vi "Bo Peep Auton.vi"() -> ()   [LabVIEW 2014]
uses:
  <vilib>/Rock Robotics/WPI/Solenoid/WPI_SolenoidValue.ctl
  <vilib>/Rock Robotics/WPI/Ultrasonic/WPI_SonarMB1010AnalogRefNum Registry Get.vi
  <vilib>/Rock Robotics/WPI/Ultrasonic/WPI_SonarMB1010AnalogGetRange.vi
  Robot Global Data.vi
  <vilib>/Rock Robotics/WPI/Solenoid/WPI_SolenoidSetEnum.vi
  <vilib>/Rock Robotics/WPI/RobotDrive/WPI_RobotDriveGetSetRefNum.vi
  <vilib>/Rock Robotics/WPI/RobotDrive/WPI_RobotDriveMecanumDrive_Cartesian.vi
panel:
  in  "Test":bool
  in  "Force state bo peep":i8
  out "Result":dbl(graph)
  out "result":dbl
  out "Destination":dbl
  out "Side Distance":dbl(graph)
  out "Front Distance":dbl(graph)
  out "Back Distance":dbl(graph)
  out "Bin Counter":i8
  out "Move?":bool
  out "Last State":i8
  out "State":i8
  out "Back Distance":dbl
  out "Front Distance":dbl
  out "Side Distance":dbl
  out "Bin found?":bool
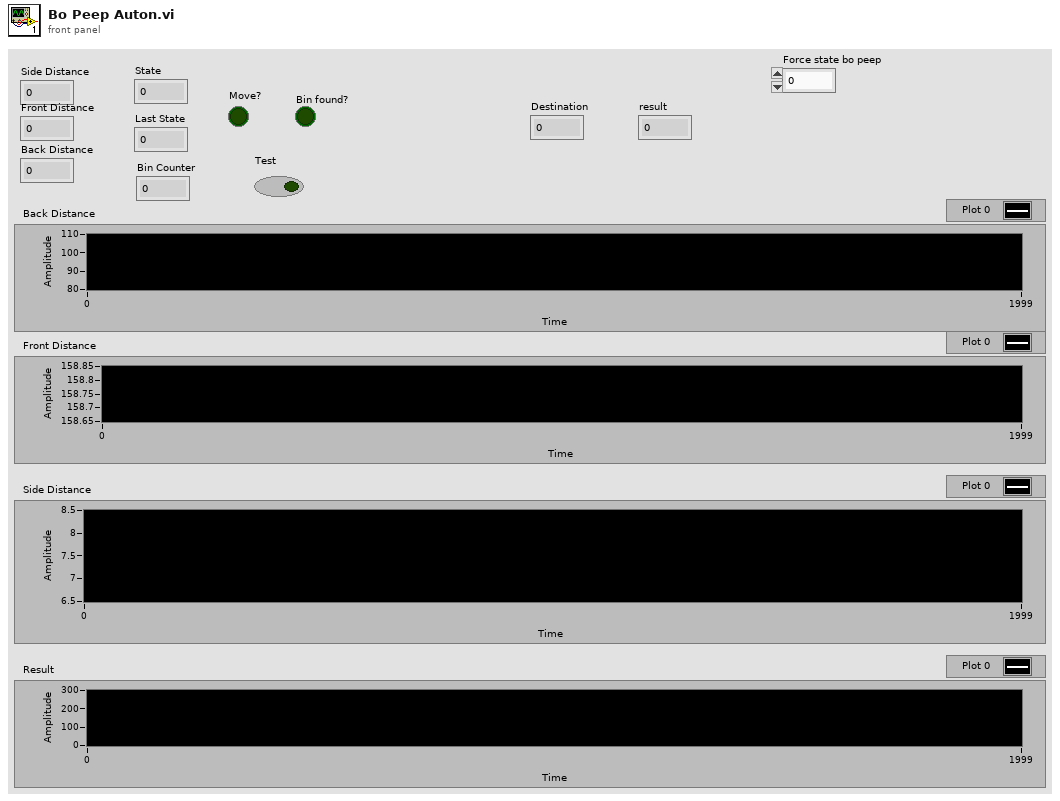
[diagram p1: front panel]
types:
  T1 = typedef "WPI_SonarMB1010AnalogDeviceRef.ctl" = cluster{"AIDeviceRef":T2, "Scaling factor (V/in)":dbl, "Average Bits":u8}
  T2 = typedef "WPI_AnalogChannelDevRef.ctl" = cluster{"DevStatus":errorcluster, "Controller":T3, "Analog Channel":T4}
  T3 = typedef "FPGA_TypedefAnalogModule.ctl" = enum16{"Controller 1"}
  T4 = typedef "FPGA_AIChannel.ctl" = enum8{"AI 0", "AI 1", "AI 2", "AI 3", "AI MXP 0", "AI MXP 1", "AI MXP 2", "AI MXP 3", "Invalid"}
  T5 = typedef "WPI_SolenoidValue.ctl" = enum16{"Off", "On", "Forward", "Reverse"}
  T6 = typedef "WPI_ServoDeviceRef.ctl" = cluster{"DeviceStatus":errorcluster, "Controller":T7, "PWM Channel":T8, "DeadBand":T9}
  T7 = typedef "FPGA_TypedefDigitalModule.ctl" = enum16{"Controller 1"}
  T8 = typedef "FPGA_DIOPWMChannel.ctl" = enum8{"PWM 0", "PWM 1", "PWM 2", "PWM 3", "PWM 4", "PWM 5", "PWM 6", "PWM 7", "PWM 8", "PWM 9", "PWM MXP 0", "PWM MXP 1", "PWM MXP 2", "PWM MXP 3", "PWM MXP 4", "PWM MXP 5", "PWM MXP 6", "PWM MXP 7", "PWM MXP 8", "PWM MXP 9", "Invalid"}
  T9 = typedef "WPI_PWMDeadband.ctl" = cluster{"Name":string, "maxPositivePwm":i32, "minPositivePwm":i32, "centerPwm":i32, "maxNegativePwm":i32, "minNegativePwm":i32, "angularRange":u16}
  T10 = typedef "WPI_MotorControlDeviceRef.ctl" = cluster{"DeviceStatus":errorcluster, "Type":T11, "PWM":cluster{"Controller":T7, "PWM Channel":T8, "DeadBand":T9}, "CAN":cluster{"Device Number":u8, "Control Mode":T12, "Semaphore":T13, "Max Vout":dbl, "TalonSRX Control Mode":T14}, "Invert":bool, "TransformRef":T15, "InvTransformRef":T15}
  T11 = typedef "WPI_MotorControlType.ctl" = enum16{"PWM", "CAN", "CANTalonSRX"}
  T12 = typedef "WPI_CANJaguar_ControlMode.ctl" = enum8{"Percent VBus", "Current", "Speed", "Position", "Voltage"}
  T13 = typedef "Semaphore RefNum" = refnum<k1>
  T14 = typedef "WPI_CANTalonSRX_APIControlMode.ctl" = enum8{"Percent VBus", "Speed", "Position", "Slave", "Unchanged / Invalid"}
  T15 = typedef "WPI_PWMTransform_ConPane.ctl" = refnum<vi>
  T16 = typedef "WPI_SolenoidDevRef.ctl" = cluster{"DevStatus":errorcluster, "Pneumatics Control Module":u8, "Forward Solenoid Channel":T17, "Reverse Solenoid Channel":T17}
  T17 = typedef "WPI_SolenoidChannel.ctl" = enum8{"Solenoid 0", "Solenoid 1", "Solenoid 2", "Solenoid 3", "Solenoid 4", "Solenoid 5", "Solenoid 6", "Solenoid 7", "Invalid"}
  T18 = typedef "WPI_CANTalonSRX_GlobalStatus.ctl" = cluster{"Applied Throttle":dbl, "Module Enabled":bool, "CAN Error":errorcluster, "Closed Loop Error":dbl, "Forward Limit Switch Closed":bool, "Reverse Limit Switch Closed":bool, "Sensor Position":dbl, "Sensor Velocity":dbl, "Current":dbl, "Sticky Fault - Over Temp":bool, "Sticky Fault - Under Voltage":bool, "Sticky Fault - Forward Limit":bool, "Sticky Fault - Reverse Limit":bool, "Sticky Fault - Forward Soft Limit":bool, "Sticky Fault - Reverse Soft Limit":bool, "Brake is Enabled":bool, "Encoder Position":dbl, "Encoder Velocity":dbl, "Encoder Index Count":dbl, "Encoder A Pin State":bool, "Encoder B Pin State":bool, "Encoder Index Pin State":bool, "Analog In":dbl, "Analog In Velocity":dbl, "Temperature (C)":dbl, "Battery Voltage":dbl}
  T19 = typedef "WPI_DigitalInputDevRef.ctl" = cluster{"DevStatus":errorcluster, "DIO Channel":T20, "Controller":T7}
  T20 = typedef "FPGA_DIOChannel.ctl" = enum8{"DIO 0", "DIO 1", "DIO 2", "DIO 3", "DIO 4", "DIO 5", "DIO 6", "DIO 7", "DIO 8", "DIO 9", "DIO MXP 0", "DIO MXP 1", "DIO MXP 2", "DIO MXP 3", "DIO MXP 4", "DIO MXP 5", "DIO MXP 6", "DIO MXP 7", "DIO MXP 8", "DIO MXP 9", "DIO MXP 10", "DIO MXP 11", "DIO MXP 12", "DIO MXP 13", "DIO MXP 14", "DIO MXP 15", "Invalid"}
  T21 = typedef "WPI_DigitalOutputDevRef.ctl" = cluster{"Controller":T7, "DIO Channel":T20, "DevStatus":errorcluster}
  T22 = typedef "WPI_RobotDriveDevRef.ctl" = cluster{"DevStatus":errorcluster, "Motors[]":T10[], "Square Inputs":bool, "Max Output":dbl}
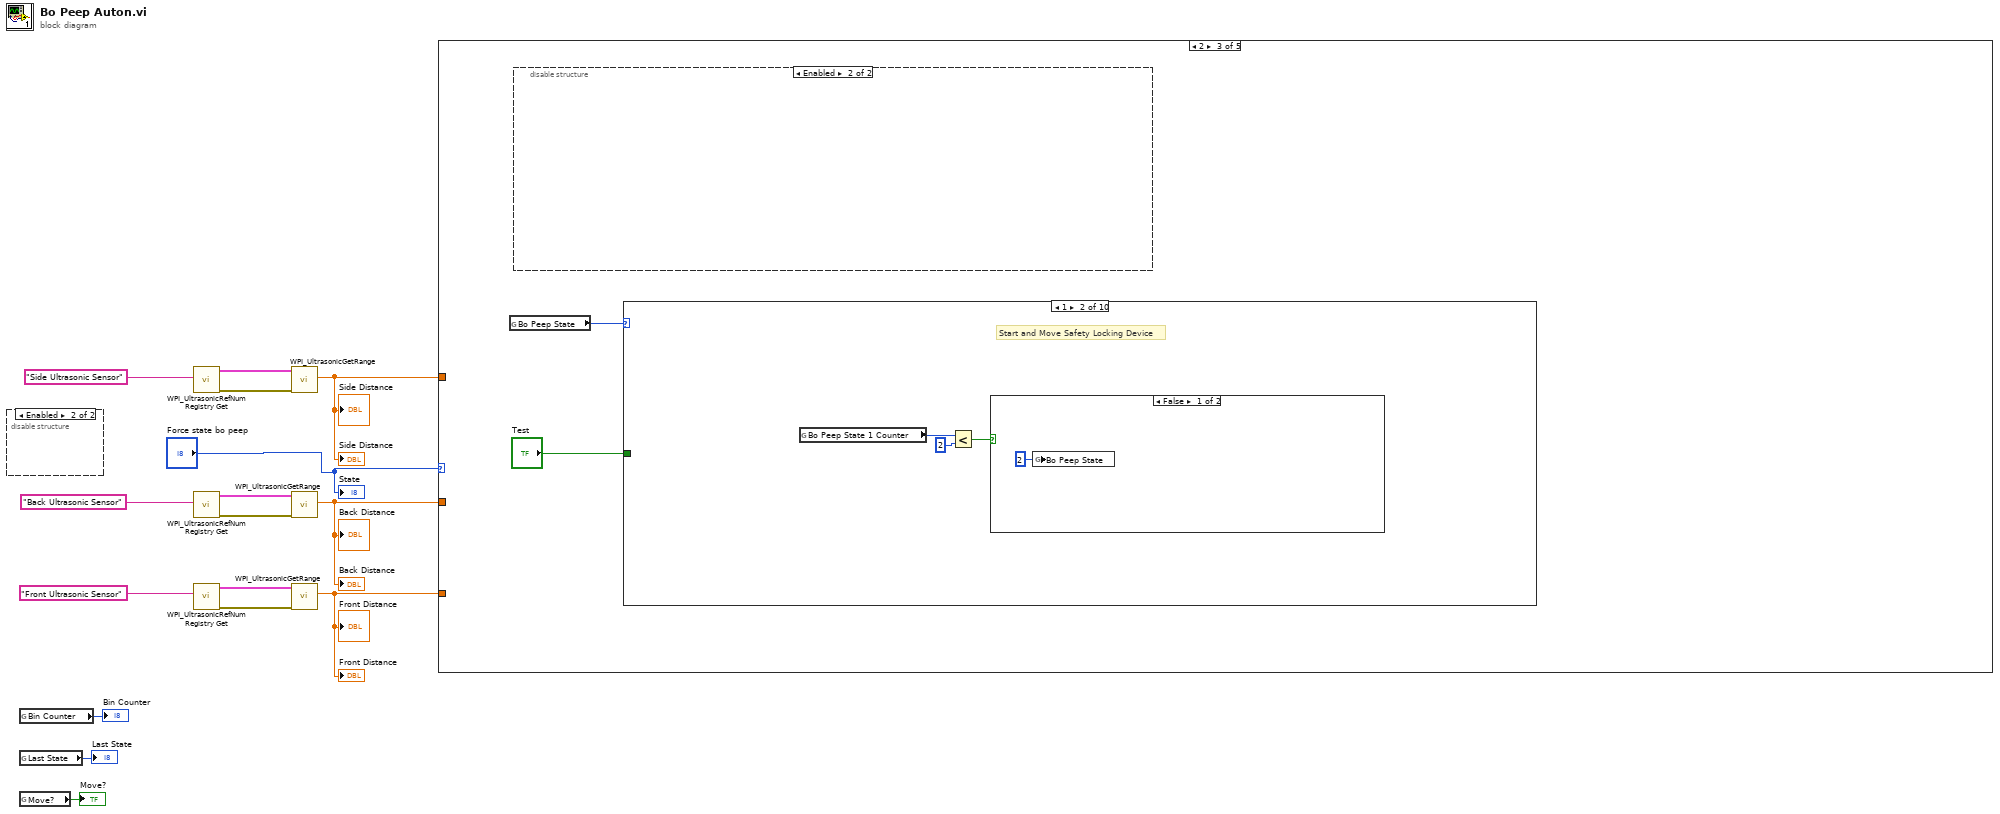
[diagram p0: block diagram]
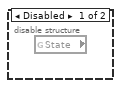
[diagram p2: hidden frame]
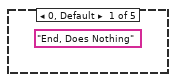
[diagram p3: hidden frame]
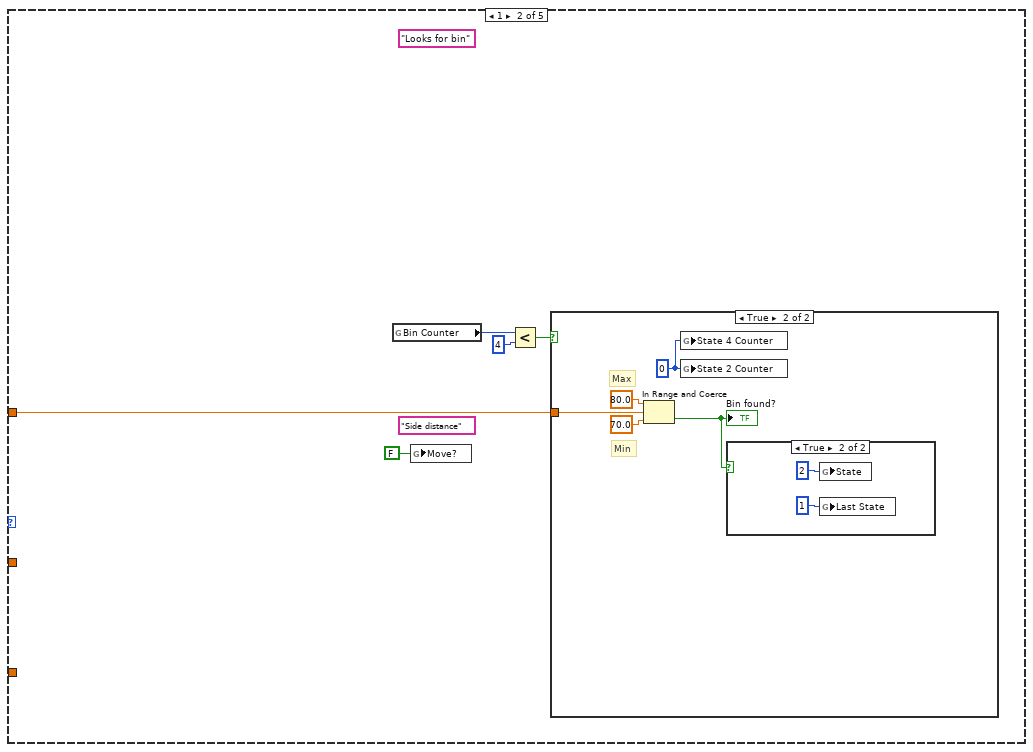
[diagram p4: hidden frame]
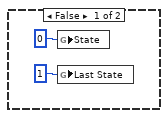
[diagram p5: hidden frame]
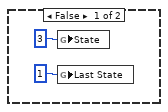
[diagram p6: hidden frame]
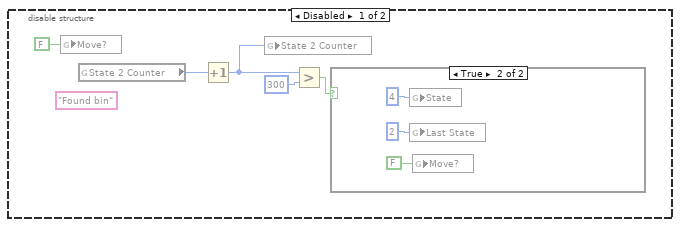
[diagram p7: hidden frame]
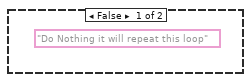
[diagram p8: hidden frame]
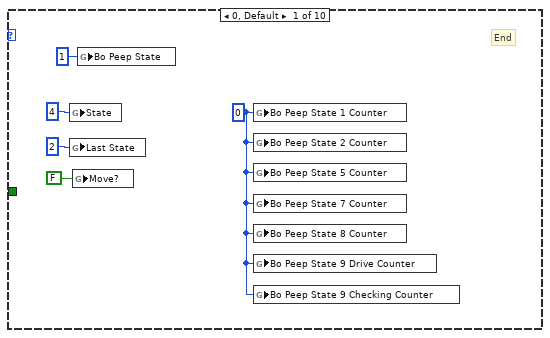
[diagram p9: hidden frame]
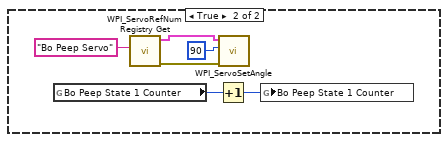
[diagram p10: hidden frame]
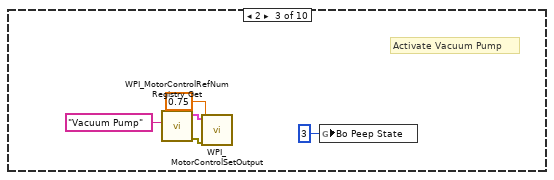
[diagram p11: hidden frame]
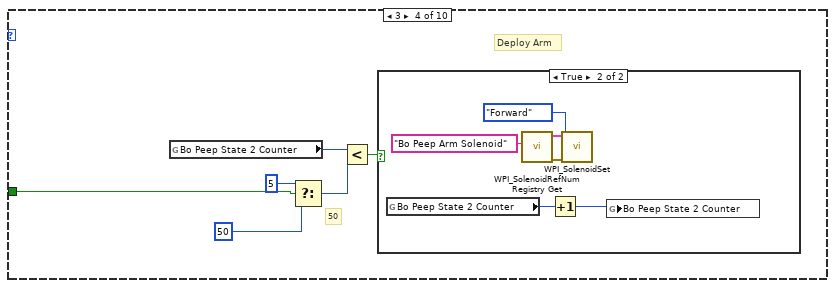
[diagram p12: hidden frame]
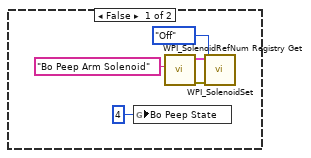
[diagram p13: hidden frame]
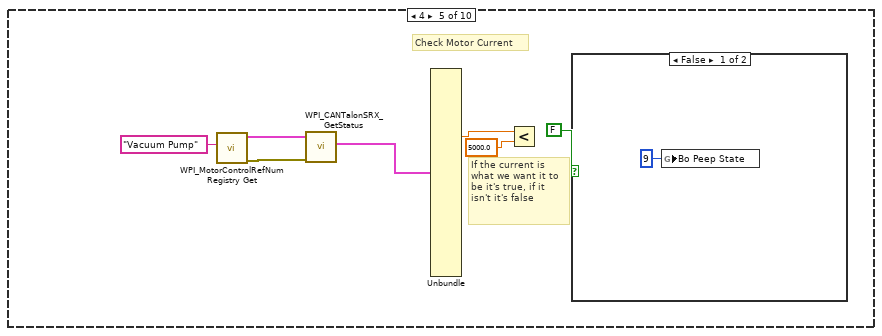
[diagram p14: hidden frame]
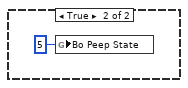
[diagram p15: hidden frame]
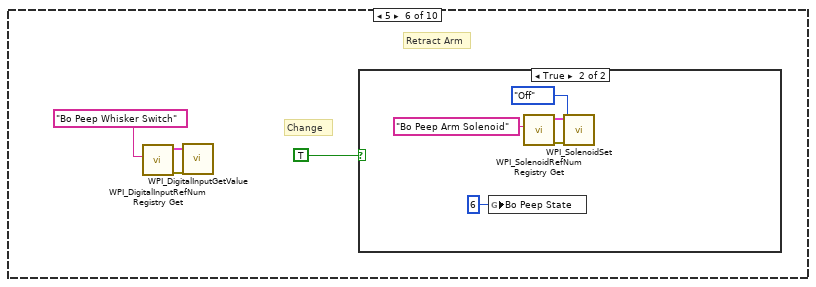
[diagram p16: hidden frame]
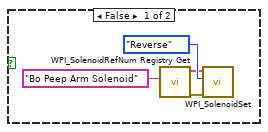
[diagram p17: hidden frame]
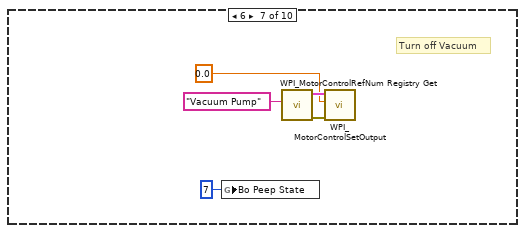
[diagram p18: hidden frame]
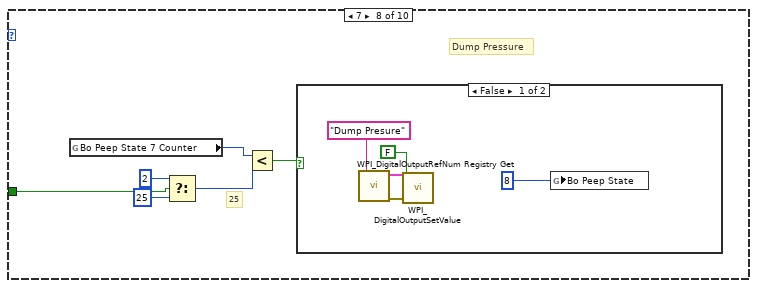
[diagram p19: hidden frame]
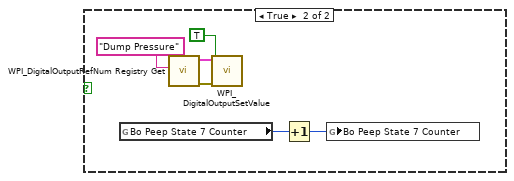
[diagram p20: hidden frame]
diagram:
  n1 = disable-structure shown="Enabled" {
    frame Disabled {
      n2 = global read "Robot Global Data.vi" "State"() -> ()  [unwired: 1 out]
    }
    frame Enabled {
    }
  }
  n3 = global read "Robot Global Data.vi" "Bin Counter"() -> (→"Bin Counter":i8)
  n4 = global read "Robot Global Data.vi" "Last State"() -> (→"Last State":i8)
  n5 = global read "Robot Global Data.vi" "Move?"() -> (→"Move?":bool)
  n6 = call-poly <vilib>:"WPI_UltrasonicRefNum Registry Get.vi"("refnum name"="Side Ultrasonic Sensor") -> ("error out"=w11:errorcluster, "SonarMB1010AnalogDevRef"=w12:T1)  [unwired: 9 in]
  n7 = call-poly <vilib>:"WPI_UltrasonicRefNum Registry Get.vi"("refnum name"="Back Ultrasonic Sensor") -> ("error out"=w8:errorcluster, "SonarMB1010AnalogDevRef"=w9:T1)  [unwired: 9 in]
  n8 = call-poly <vilib>:"WPI_UltrasonicRefNum Registry Get.vi"("refnum name"="Front Ultrasonic Sensor") -> ("error out"=w15:errorcluster, "SonarMB1010AnalogDevRef"=w16:T1)  [unwired: 9 in]
  n9 = call-poly <vilib>:"WPI_UltrasonicGetRange.vi"("error in"=w11, "SonarMB1010AnalogDevRef"=w12) -> ("Distance"=w3:dbl)  [unwired: 7 in, 2 out]
  "Side Distance" <- w3
  "Side Distance" <- w3
  n10 = call-poly <vilib>:"WPI_UltrasonicGetRange.vi"("error in"=w8, "SonarMB1010AnalogDevRef"=w9) -> ("Distance"=w2:dbl)  [unwired: 7 in, 2 out]
  "Back Distance" <- w2
  "Back Distance" <- w2
  n11 = call-poly <vilib>:"WPI_UltrasonicGetRange.vi"("error in"=w15, "SonarMB1010AnalogDevRef"=w16) -> ("Distance"=w4:dbl)  [unwired: 7 in, 2 out]
  "Front Distance" <- w4
  "Front Distance" <- w4
  n12 = case shown="2" "Force state bo peep" {
    tunnel: w3 -> [_ w21 _ _ _]
    tunnel: w4 -> [_ _ _ _ w175]
    tunnel: w2 -> [_ _ _ _ w174]
    frame 0, Default {
      (unwired) "End, Does Nothing"
    }
    frame 1 {
      (unwired) "Side distance"
      (unwired) "Looks for bin"
      n13 = global read "Robot Global Data.vi" "Bin Counter"() -> (w19:i8)
      n14 = global write "Robot Global Data.vi" "Move?"(FALSE ("Move?")) -> ()
      n15 = Less?(x=w19, y=i8 4) -> (x < y?=w20:bool)
      n16 = case shown="True" w20 {
        tunnel: w21 -> [_ w25]
        frame False {
          n17 = global write "Robot Global Data.vi" "State"(i8 0 ("State")) -> ()
          n18 = global write "Robot Global Data.vi" "Last State"(i8 1 ("Last State")) -> ()
        }
        frame True {
          w24 = i16 0 ("State 2 Counter")
          # "Max"
          # "Min"
          n19 = In Range and Coerce(upper limit=80.0, x=w25, lower limit=70.0) -> (In Range?=w26:bool)  [unwired: 1 out]
          "Bin found?" <- w26
          n20 = global write "Robot Global Data.vi" "State 4 Counter"(w24) -> ()
          n21 = global write "Robot Global Data.vi" "State 2 Counter"(w24) -> ()
          n22 = case shown="True" w26 {
            frame False {
              n23 = global write "Robot Global Data.vi" "State"(i8 3 ("State")) -> ()
              n24 = global write "Robot Global Data.vi" "Last State"(i8 1 ("Last State")) -> ()
            }
            frame True {
              n25 = global write "Robot Global Data.vi" "State"(i8 2 ("State")) -> ()
              n26 = global write "Robot Global Data.vi" "Last State"(i8 1 ("Last State")) -> ()
            }
          }
        }
      }
    }
    frame 2 {
      n27 = global read "Robot Global Data.vi" "Bo Peep State"() -> (w34:i8)
      n28 = disable-structure shown="Enabled" {
        frame Disabled {
          (unwired) "Found bin"
          n29 = global write "Robot Global Data.vi" "Move?"(FALSE) -> ()
          n30 = global read "Robot Global Data.vi" "State 2 Counter"() -> (w38:i16)
          n31 = Increment(x=w38) -> (x+1=w37:i16)
          n32 = global write "Robot Global Data.vi" "State 2 Counter"(w37) -> ()
          n33 = Greater?(x=w37, y=i16 300) -> (0:w35:bool)
          n34 = case shown="True" w35 {
            frame False {
              (unwired) "Do Nothing it will repeat this loop"
            }
            frame True {
              n35 = global write "Robot Global Data.vi" "State"(i8 4 ("State")) -> ()
              n36 = global write "Robot Global Data.vi" "Last State"(i8 2 ("Last State")) -> ()
              n37 = global write "Robot Global Data.vi" "Move?"(FALSE) -> ()
            }
          }
        }
        frame Enabled {
        }
      }
      n38 = case shown="1" w34 {
        tunnel: "Test" -> [_ _ _ w63 _ _ _ w108 _ _]
        frame 0, Default {
          w44 = i8 0 ("Bo Peep State 1 Counter")
          # "End"
          n39 = global write "Robot Global Data.vi" "State"(i8 4 ("State")) -> ()
          n40 = global write "Robot Global Data.vi" "Last State"(i8 2 ("Last State")) -> ()
          n41 = global write "Robot Global Data.vi" "Move?"(FALSE) -> ()
          n42 = global write "Robot Global Data.vi" "Bo Peep State"(i8 1 ("Bo Peep State")) -> ()
          n43 = global write "Robot Global Data.vi" "Bo Peep State 1 Counter"(w44) -> ()
          n44 = global write "Robot Global Data.vi" "Bo Peep State 2 Counter"(w44) -> ()
          n45 = global write "Robot Global Data.vi" "Bo Peep State 5 Counter"(w44) -> ()
          n46 = global write "Robot Global Data.vi" "Bo Peep State 7 Counter"(w44) -> ()
          n47 = global write "Robot Global Data.vi" "Bo Peep State 8 Counter"(w44) -> ()
          n48 = global write "Robot Global Data.vi" "Bo Peep State 9 Drive Counter"(w44) -> ()
          n49 = global write "Robot Global Data.vi" "Bo Peep State 9 Checking Counter"(w44) -> ()
        }
        frame 1 {
          # "Start and Move Safety Locking Device"
          n50 = global read "Robot Global Data.vi" "Bo Peep State 1 Counter"() -> (w50:i8)
          n51 = Less?(x=w50, y=i8 2) -> (x < y?=w48:bool)
          n52 = case shown="False" w48 {
            frame False {
              n53 = global write "Robot Global Data.vi" "Bo Peep State"(i8 2 ("Bo Peep State")) -> ()
            }
            frame True {
              n54 = global read "Robot Global Data.vi" "Bo Peep State 1 Counter"() -> (w56:i8)
              n55 = call <vilib>:"WPI_ServoRefNum Registry Get.vi"("refnum name"="Bo Peep Servo") -> ("error out"=w53:errorcluster, "ServoDeviceRef"=w54:T6)  [unwired: 9 in]
              n56 = Increment(x=w56) -> (x+1=w57:i8)
              n57 = call <vilib>:"WPI_ServoSetAngle.vi"("error in (no error)"=w53, "Angle"=90, "ServoDeviceRef"=w54) -> ()  [unwired: 7 in, 2 out]
              n58 = global write "Robot Global Data.vi" "Bo Peep State 1 Counter"(w57) -> ()
            }
          }
        }
        frame 2 {
          # "Activate Vacuum Pump"
          n59 = call <vilib>:"WPI_MotorControlRefNum Registry Get.vi"("refnum name"="Vacuum Pump") -> ("error out"=w62:errorcluster, "MotorControlDevRef"=w61:T10)  [unwired: 9 in]
          n60 = call <vilib>:"WPI_MotorControlSetOutput.vi"("error in (no error)"=w62, "Output"=0.75, "MotorControlDevRef"=w61) -> ()  [unwired: 6 in, 3 out]
          n61 = global write "Robot Global Data.vi" "Bo Peep State"(i8 3 ("Bo Peep State")) -> ()
        }
        frame 3 {
          # "50"
          # "Deploy Arm"
          n62 = global read "Robot Global Data.vi" "Bo Peep State 2 Counter"() -> (w67:i8)
          n63 = Select(t=i8 5, s=w63, f=i8 50 ("y")) -> (s? t:f=w66:i8)
          n64 = Less?(x=w67, y=w66) -> (x < y?=w68:bool)
          n65 = case shown="True" w68 {
            frame False {
              n66 = global write "Robot Global Data.vi" "Bo Peep State"(i8 4 ("Bo Peep State")) -> ()
              n67 = call <vilib>:"WPI_SolenoidRefNum Registry Get.vi"("refnum name"="Bo Peep Arm Solenoid") -> ("error out"=w70:errorcluster, "SolenoidDevRef"=w71:T16)  [unwired: 9 in]
              n68 = call-poly <vilib>:"WPI_SolenoidSet.vi"("error in (no error)"=w70, "Value"=WPI_SolenoidValue."Off", "SolenoidDevRef"=w71) -> ()  [unwired: 7 in, 2 out]
            }
            frame True {
              n69 = global read "Robot Global Data.vi" "Bo Peep State 2 Counter"() -> (w75:i8)
              n70 = call <vilib>:"WPI_SolenoidRefNum Registry Get.vi"("refnum name"="Bo Peep Arm Solenoid") -> ("error out"=w77:errorcluster, "SolenoidDevRef"=w78:T16)  [unwired: 9 in]
              n71 = Increment(x=w75) -> (x+1=w74:i8)
              n72 = call-poly <vilib>:"WPI_SolenoidSet.vi"("error in (no error)"=w77, "Value"=WPI_SolenoidValue."Forward", "SolenoidDevRef"=w78) -> ()  [unwired: 7 in, 2 out]
              n73 = global write "Robot Global Data.vi" "Bo Peep State 2 Counter"(w74) -> ()
            }
          }
        }
        frame 4 {
          # "If the current is what we want it to be it's true, if it isn't it's false"
          # "Check Motor Current"
          n74 = call <vilib>:"WPI_MotorControlRefNum Registry Get.vi"("refnum name"="Vacuum Pump") -> ("error out"=w85:errorcluster, "MotorControlDevRef"=w84:T10)  [unwired: 9 in]
          n75 = call <vilib>:"WPI_CANTalonSRX_GetStatus.vi"("error in (no error)"=w85, "CAN Talon SRX Ref"=w84) -> ("Talon SRX Status"=w83:T18)  [unwired: 7 in, 2 out]
          n76 = Unbundle(w83) -> ("Current"=w82:dbl)  [unwired: 25 out]
          n77 = Less?(x=w82, y=5000.0) -> ()  [unwired: 1 out]
          n78 = case shown="False" FALSE {
            frame False {
              n79 = global write "Robot Global Data.vi" "Bo Peep State"(i8 9 ("Bo Peep State")) -> ()
            }
            frame True {
              n80 = global write "Robot Global Data.vi" "Bo Peep State"(i8 5 ("Bo Peep State")) -> ()
            }
          }
        }
        frame 5 {
          # "Change"
          # "Retract Arm"
          n81 = call <vilib>:"WPI_DigitalInputRefNum Registry Get.vi"("refnum name"="Bo Peep Whisker Switch") -> ("error out"=w91:errorcluster, "DigitalInputDevRef"=w90:T19)  [unwired: 9 in]
          n82 = call <vilib>:"WPI_DigitalInputGetValue.vi"("error in (no error)"=w91, "DigitalInputDevRef"=w90) -> ()  [unwired: 7 in, 3 out]
          n83 = case shown="True" TRUE {
            frame False {
              n84 = call <vilib>:"WPI_SolenoidRefNum Registry Get.vi"("refnum name"="Bo Peep Arm Solenoid") -> ("error out"=w94:errorcluster, "SolenoidDevRef"=w95:T16)  [unwired: 9 in]
              n85 = call-poly <vilib>:"WPI_SolenoidSet.vi"("error in (no error)"=w94, "Value"=WPI_SolenoidValue."Reverse", "SolenoidDevRef"=w95) -> ()  [unwired: 7 in, 2 out]
            }
            frame True {
              n86 = global write "Robot Global Data.vi" "Bo Peep State"(i8 6 ("Bo Peep State")) -> ()
              n87 = call <vilib>:"WPI_SolenoidRefNum Registry Get.vi"("refnum name"="Bo Peep Arm Solenoid") -> ("error out"=w98:errorcluster, "SolenoidDevRef"=w99:T16)  [unwired: 9 in]
              n88 = call-poly <vilib>:"WPI_SolenoidSet.vi"("error in (no error)"=w98, "Value"=WPI_SolenoidValue."Off", "SolenoidDevRef"=w99) -> ()  [unwired: 7 in, 2 out]
            }
          }
        }
        frame 6 {
          # "Turn off Vacuum"
          n89 = global write "Robot Global Data.vi" "Bo Peep State"(i8 7 ("Bo Peep State")) -> ()
          n90 = call <vilib>:"WPI_MotorControlRefNum Registry Get.vi"("refnum name"="Vacuum Pump") -> ("error out"=w106:errorcluster, "MotorControlDevRef"=w105:T10)  [unwired: 9 in]
          n91 = call <vilib>:"WPI_MotorControlSetOutput.vi"("error in (no error)"=w106, "Output"=0.0, "MotorControlDevRef"=w105) -> ()  [unwired: 6 in, 3 out]
        }
        frame 7 {
          # "25"
          # "Dump Pressure"
          n92 = global read "Robot Global Data.vi" "Bo Peep State 7 Counter"() -> (w112:i8)
          n93 = Select(t=i8 2, s=w108, f=i8 25) -> (s? t:f=w110:i8)
          n94 = Less?(x=w112, y=w110) -> (x < y?=w111:bool)
          n95 = case shown="False" w111 {
            frame False {
              n96 = call <vilib>:"WPI_DigitalOutputRefNum Registry Get.vi"("refnum name"="Dump Presure") -> ("error out"=w117:errorcluster, "DigitalOutputDevRef"=w116:T21)  [unwired: 9 in]
              n97 = call <vilib>:"WPI_DigitalOutputSetValue.vi"("error in (no error)"=w117, "Value"=FALSE, "DigitalOutputDevRef"=w116) -> ()  [unwired: 7 in, 2 out]
              n98 = global write "Robot Global Data.vi" "Bo Peep State"(i8 8 ("Bo Peep State 1 Counter")) -> ()
            }
            frame True {
              n99 = global read "Robot Global Data.vi" "Bo Peep State 7 Counter"() -> (w119:i8)
              n100 = call <vilib>:"WPI_DigitalOutputRefNum Registry Get.vi"("refnum name"="Dump Pressure") -> ("error out"=w123:errorcluster, "DigitalOutputDevRef"=w122:T21)  [unwired: 9 in]
              n101 = call <vilib>:"WPI_DigitalOutputSetValue.vi"("error in (no error)"=w123, "Value"=TRUE, "DigitalOutputDevRef"=w122) -> ()  [unwired: 7 in, 2 out]
              n102 = Increment(x=w119) -> (x+1=w120:i8)
              n103 = global write "Robot Global Data.vi" "Bo Peep State 7 Counter"(w120) -> ()
            }
          }
        }
        frame 8 {
          # "Move Safety Locking Device to Closed Position"
          n104 = global read "Robot Global Data.vi" "Bo Peep State 8 Counter"() -> (w126:i8)
          n105 = Less?(x=w126, y=i8 2) -> (x < y?=w124:bool)
          n106 = case shown="True" w124 {
            frame False {
              n107 = global write "Robot Global Data.vi" "Bo Peep State"(i8 0 ("Bo Peep State")) -> ()
            }
            frame True {
              n108 = global read "Robot Global Data.vi" "Bo Peep State 8 Counter"() -> (w132:i8)
              n109 = call <vilib>:"WPI_ServoRefNum Registry Get.vi"("refnum name"="Bo Peep Servo") -> ("error out"=w129:errorcluster, "ServoDeviceRef"=w130:T6)  [unwired: 9 in]
              n110 = Increment(x=w132) -> (x+1=w133:i8)
              n111 = call <vilib>:"WPI_ServoSetAngle.vi"("error in (no error)"=w129, "Angle"=0, "ServoDeviceRef"=w130) -> ()  [unwired: 7 in, 2 out]
              n112 = global write "Robot Global Data.vi" "Bo Peep State 8 Counter"(w133) -> ()
            }
          }
        }
        frame 9 {
          n113 = global read "Robot Global Data.vi" "Bo Peep State 9 Checking Counter"() -> (w136:i8)
          n114 = Less?(x=w136, y=i8 5) -> (x < y?=w134:bool)
          n115 = case shown="True" w134 {
            frame False {
              n116 = global write "Robot Global Data.vi" "Bo Peep State"(i8 0 ("Bo Peep State")) -> ()
            }
            frame True {
              n117 = global read "Robot Global Data.vi" "Bo Peep State 9 Drive Counter"() -> (w140:i8)
              n118 = global read "Robot Global Data.vi" "Bo Peep State 9 Checking Counter"() -> (w142:i8)
              n119 = Less?(x=w140, y=i8 5) -> (x < y?=w138:bool)
              n120 = Increment(x=w142) -> (x+1=w141:i8)
              n121 = case shown="True" w138 {
                frame False {
                  n122 = global write "Robot Global Data.vi" "Bo Peep State"(i8 4 ("Bo Peep State")) -> ()
                  n123 = call <vilib>:"WPI_RobotDriveRefNum Registry Get.vi"("refnum name"="Four Motors") -> ("error out"=w148:errorcluster, "RobotDriveDevRef"=w149:T22)  [unwired: 9 in]
                  n124 = global write "Robot Global Data.vi" "Bo Peep State 9 Drive Counter"(i8 0 ("Bo Peep State 9 Drive Counter")) -> ()
                  n125 = call-poly <vilib>:"WPI_RobotDriveHolonomicDrive.vi"("Rotation"=0.0, "error in (no error)"=w148, "Y"=0.0, "X"=0.0, "RobotDriveDevRef"=w149) -> ()  [unwired: 4 in, 3 out]
                }
                frame True {
                  # ".5"
                  n126 = global read "Robot Global Data.vi" "Bo Peep State 9 Drive Counter"() -> (w154:i8)
                  n127 = call <vilib>:"WPI_RobotDriveRefNum Registry Get.vi"("refnum name"="Four Motors") -> ("error out"=w156:errorcluster, "RobotDriveDevRef"=w157:T22)  [unwired: 9 in]
                  n128 = Increment(x=w154) -> (x+1=w153:i8)
                  n129 = global write "Robot Global Data.vi" "Bo Peep State 9 Drive Counter"(w153) -> ()
                  n130 = call-poly <vilib>:"WPI_RobotDriveHolonomicDrive.vi"("Rotation"=0.0, "error in (no error)"=w156, "Y"=0.0, "X"=0.0, "RobotDriveDevRef"=w157) -> ()  [unwired: 4 in, 3 out]
                }
              }
              n131 = global write "Robot Global Data.vi" "Bo Peep State 9 Checking Counter"(w141) -> ()
            }
          }
        }
      }
    }
    frame 3 {
      (unwired) "Didn't Find Bin"
      n132 = global read "Robot Global Data.vi" "State 3 Counter"() -> (w162:i16)
      n133 = Increment(x=w162) -> (x+1=w161:i16)
      n134 = global write "Robot Global Data.vi" "State 3 Counter"(w161) -> ()
      n135 = Greater?(x=w161, y=i16 5) -> (0:w159:bool)
      n136 = case shown="True" w159 {
        frame False {
          n137 = global write "Robot Global Data.vi" "State"(i8 1 ("State")) -> ()
          n138 = global write "Robot Global Data.vi" "Last State"(i8 3 ("State")) -> ()
        }
        frame True {
          n139 = global write "Robot Global Data.vi" "State"(i8 4 ("State")) -> ()
          n140 = global write "Robot Global Data.vi" "Last State"(i8 3 ("State")) -> ()
        }
      }
    }
    frame 4 {
      w168 = 17.5
      w181 = 288.0 ("y")
      w177 = 0.0 ("lower limit")
      w176 = 180.0 ("upper limit")
      (unwired) "Drive x Distance"
      # "FIND ROBOT WIDTH AND INTEGRATE IT PLEASE"
      n141 = global read "Robot Global Data.vi" "Bin Counter"() -> (w185:i8)
      n142 = In Range and Coerce(upper limit=w176, x=w174, lower limit=w177) -> (In Range?=w169:bool)  [unwired: 1 out]
      n143 = In Range and Coerce(upper limit=w176, x=w175, lower limit=w177) -> (In Range?=w172:bool)  [unwired: 1 out]
      n144 = Not(x=w169) -> (.not. x?=w170:bool)
      n145 = And(x=w172, y=w170) -> (x .and. y?=w180:bool)
      n146 = And(x=w169, y=w172) -> (x .and. y?=w178:bool)
      n147 = case shown="True" w178 {
        tunnel: w174 -> [_ w202]
        tunnel: w175 -> [_ w200]
        tunnel: w181 -> [_ w203]
        tunnel: [0.0 w197] -> w182
        frame False {
        }
        frame True {
          n148 = Add(x=w202, y=w203) -> (x+y=w201:dbl)
          n149 = Subtract(x=w201, y=w200) -> (x-y=w199:dbl)
          n150 = Divide(x=w199, y=2.0) -> (x/y=w197:dbl)
        }
      }
      n151 = case shown="True" w180 {
        tunnel: w181 -> [_ w191]
        tunnel: w175 -> [_ w190]
        tunnel: [0.0 w187] -> w184
        tunnel: w168 -> [_ w188]
        frame False {
        }
        frame True {
          n152 = Subtract(x=w191, y=w190) -> (x-y=w189:dbl)
          n153 = Subtract(x=w189, y=w188) -> (x-y=w187:dbl)
        }
      }
      n154 = Not(x=w172) -> (.not. x?=w171:bool)
      n155 = And(x=w169, y=w171) -> (x .and. y?=w179:bool)
      n156 = case shown="True" w179 {
        tunnel: w174 -> [_ w194]
        tunnel: [0.0 w193] -> w183
        tunnel: w168 -> [_ w195]
        frame False {
        }
        frame True {
          n157 = Add(x=w194, y=w195) -> (x+y=w193:dbl)
        }
      }
      n158 = Compound Arithmetic op=ADD(w182, w183, w184) -> (w173:dbl)
      "result" <- w173
      "Result" <- w173
      n159 = case shown="1" w185 {
        tunnel: w173 -> [_ w206 w215 w224]
        tunnel: [0.0 ("y") w205 w214 w223] -> w167
        frame 0, Default {
        }
        frame 1 {
          w205 = 108.5 ("y")
          n160 = Less?(x=w206, y=w205) -> (x < y?=w207:bool)
          n161 = case shown="False" w207 {
            frame False {
              n162 = global read "Robot Global Data.vi" "Bin Counter"() -> (w209:i8)
              n163 = global write "Robot Global Data.vi" "Last State"(i8 4 ("Last State")) -> ()
              n164 = global write "Robot Global Data.vi" "State"(i8 1 ("State")) -> ()
              n165 = global write "Robot Global Data.vi" "Move?"(FALSE) -> ()
              n166 = Increment(x=w209) -> (x+1=w208:i8)
              n167 = global write "Robot Global Data.vi" "Bin Counter"(w208) -> ()
            }
            frame True {
              n168 = global write "Robot Global Data.vi" "Move?"(TRUE) -> ()
            }
          }
        }
        frame 2 {
          w214 = 183.0 ("y")
          n169 = Less?(x=w215, y=w214) -> (x < y?=w216:bool)
          n170 = case shown="True" w216 {
            frame False {
              n171 = global read "Robot Global Data.vi" "Bin Counter"() -> (w218:i8)
              n172 = global write "Robot Global Data.vi" "Last State"(i8 4 ("Last State")) -> ()
              n173 = global write "Robot Global Data.vi" "State"(i8 1 ("State")) -> ()
              n174 = global write "Robot Global Data.vi" "Move?"(FALSE) -> ()
              n175 = Increment(x=w218) -> (x+1=w217:i8)
              n176 = global write "Robot Global Data.vi" "Bin Counter"(w217) -> ()
            }
            frame True {
              n177 = global write "Robot Global Data.vi" "Move?"(TRUE) -> ()
            }
          }
        }
        frame 3 {
          w223 = 229.0 ("y")
          n178 = Less?(x=w224, y=w223) -> (x < y?=w225:bool)
          n179 = case shown="False" w225 {
            frame False {
              n180 = global read "Robot Global Data.vi" "Bin Counter"() -> (w227:i8)
              n181 = global write "Robot Global Data.vi" "Last State"(i8 4 ("Last State")) -> ()
              n182 = global write "Robot Global Data.vi" "State"(i8 1 ("State")) -> ()
              n183 = global write "Robot Global Data.vi" "Move?"(FALSE) -> ()
              n184 = Increment(x=w227) -> (x+1=w226:i8)
              n185 = global write "Robot Global Data.vi" "Bin Counter"(w226) -> ()
            }
            frame True {
              n186 = global write "Robot Global Data.vi" "Move?"(TRUE) -> ()
            }
          }
        }
      }
      "Destination" <- w167
      n187 = call "Distance Drive.vi"("Destination"=w167, "Location"=w173) -> ()  [unwired: 10 in]
    }
  }
  "State" <- "Force state bo peep"
